vi "Read Machine Component Models.vi"(11 "名称或相对路径":string="UserDefine.ini") -> (3 "All Message":string[][](array[string]) caption="所有行")   [LabVIEW 2017]
uses:
  Global System.vi
  <vilib>/Utility/file.llb/Read From Spreadsheet File (string).vi
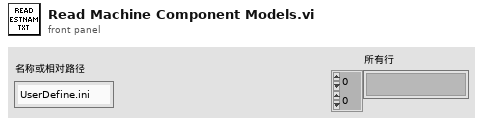
[diagram p1: front panel]
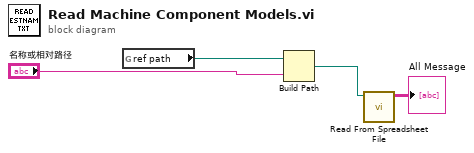
[diagram p0: block diagram]
diagram:
  n1 = global read "Global System.vi" "ref path"() -> (w4:path)
  n2 = Build Path(base path=w4, name or relative path="名称或相对路径") -> (appended path=w2:path)
  n3 = call-poly <vilib>:"Read From Spreadsheet File.vi"("file path (dialog if empty)"=w2) -> ("all rows"=→"All Message":string[][])  [unwired: 6 in, 4 out]
